vi "connection_screen.vi"(4 "error in (no error)":errorcluster, 6 "remote port":u16 max=0, 7 "address":string) -> (0 "error out":errorcluster, 3 "connection ID":refnum<k5>)   [LabVIEW 2015]
doc: "Use this template to build a PDA VI for Pocket PC 2002 devices or emulators."
panel:
  out "status":string
  in  "Cancel":bool
  in  "OK":bool
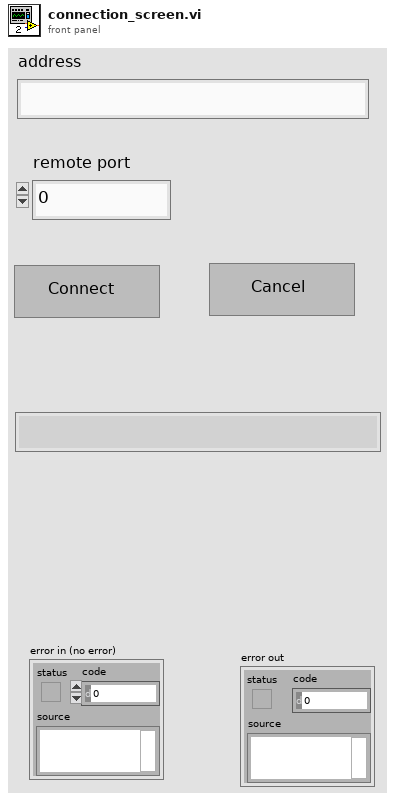
[diagram p1: front panel]
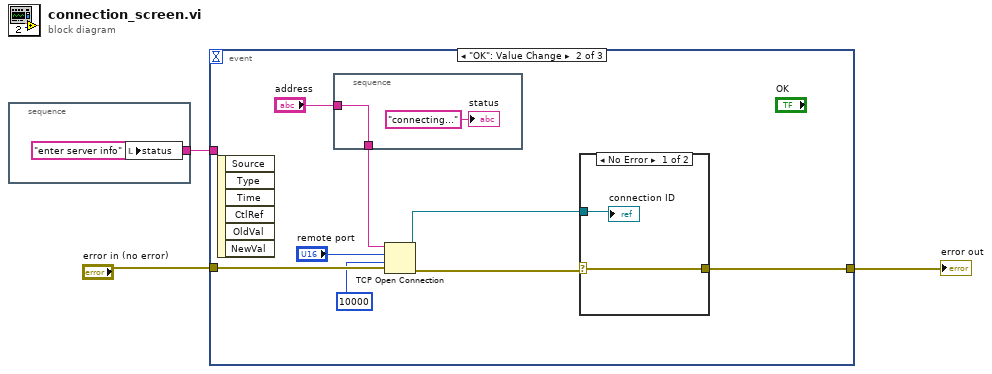
[diagram p0: block diagram]
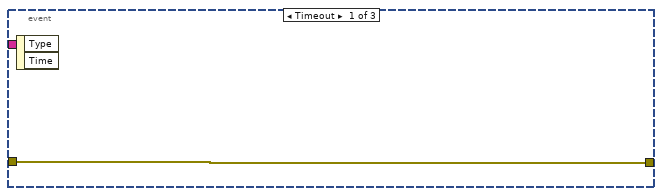
[diagram p2: hidden frame]
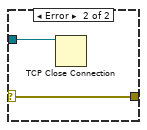
[diagram p3: hidden frame]
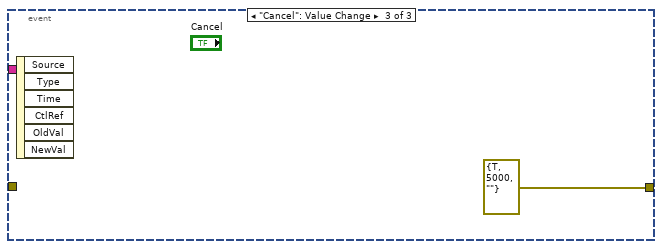
[diagram p4: hidden frame]
diagram:
  n1 = stacked-sequence {
    tunnel: [w4] -> w1
    frame #0 {
      w4 = "enter server info" ("status")
      n2 = local write "status"(w4) -> ()
    }
  }
  n3 = event shown="[1] \"OK\": Value Change" {
    selector: _ -> [_ _ _]
    dyn-events: _ -> [_ _ _]
    timeout: _ -> [_ _ _]
    tunnel: [w5 w10 errorcluster {"status"=TRUE, "code"=5000, "source"=""}] -> w2
    tunnel: "error in (no error)" -> [w5 w13 _]
    tunnel: w1 -> [_ _ _]
    event Timeout {
      n4 = event-data() -> ()  [unwired: 1 in, 2 out]
    }
    event "OK": Value Change {
      n5 = event-data() -> ()  [unwired: 1 in, 6 out]
      n6 = stacked-sequence {
        tunnel: "address" -> [w14]
        tunnel: [w14] -> w8
        frame #0 {
          "status" <- "connecting..." ("status")
        }
      }
      n7 = TCP Open Connection(address=w8, remote port or service name="remote port", timeout ms (60000)=10000, error in (no error)=w13) -> (connection ID=w6:refnum<k5>, error out=w7:errorcluster)  [unwired: 1 in]
      n8 = case shown="No Error" w7 {
        selector: w7 -> [w17 w19]
        tunnel: [w17 w19] -> w10
        tunnel: w6 -> [w16 w18]
        frame No Error {
          "connection ID" <- w16
        }
        frame Error {
          n9 = TCP Close Connection(connection ID=w18) -> ()  [unwired: 2 in, 2 out]
        }
      }
    }
    event "Cancel": Value Change {
      n10 = event-data() -> ()  [unwired: 1 in, 6 out]
    }
  }
  "error out" <- w2
